vi "Field vs Slow IV v2.1.vi"() -> ()   [LabVIEW 2024]
uses:
  <vilib>/Utility/file.llb/Write Delimited Spreadsheet (DBL).vi
panel:
  in  "Tab Control 2":enum32{"cRIO", "Lockin", "Plot 2", "Plot 3"}(tab)
  out "I vs AI":cluster{"Y":dbl[], "Y":dbl[]}[](graph)
  out "Name 0":string="DC Voltage V"
  out "I vs R":cluster{"Y":dbl[], "Y":dbl[]}[](graph)
  out "Name 1":string="DC current uA"
  out "Name 2":string="dV V"
  out "Name 3":string="dI uA"
  in  "Tab Control":T1(tab)=enum."Data log and Status"
  in  "cRIO IP":string="//172.22.11.2"
  in  "Reading Average times":i32=100
  in  "Current Start uA":dbl=-1.5
  in  "Current Range uA":dbl=3.0
  in  "Current Step uA":dbl=0.005
  in  "Current output Scale factor":dbl=1.0
  in  "Ramp type":string(combo)="Range"
  in  "Ramp up first T":bool=TRUE
  in  "AO Channel":string(combo)="AO0"
  in  "Delay Time s":dbl=0.1 caption="Delay Time (s)"
  in  "Channel name 0":string(combo)="DC Voltage V"
  in  "Scale factor0":dbl=0.0001
  in  "Chan 1":bool=TRUE
  in  "Channel name 1":string(combo)="DC current uA"
  in  "Scale factor1":dbl=1.0
  in  "Chan 2":bool
  in  "Channel name 2":string(combo)="dV V"
  in  "Scale factor2":dbl=1.0
  in  "Chan 3":bool
  in  "Channel name 3":string(combo)="dI uA"
  in  "Scale factor3":dbl=1.0
  in  "Lockin Chan name 1":string(combo)="Voltage mV"
  in  "Lockin Chan name 2":string(combo)="Current mV"
  in  "Use Lockin":bool
  in  "Lockin 1":bool
  in  "Lockin 2":bool
  in  "Lockin address 1":string="GPIB0::8::INSTR"
  in  "Lockin address 2":string="GPIB0::9::INSTR"
  in  "Lockin Status":string
  in  "Contour plot folder":path=path "C:/Users/gyue/Desktop/20230814 Soorya devices"
  in  "Book name":string="book793"
  in  "Current VI path":path=path "C:/Users/gyue/Desktop/General-Measurement/cRIO related/Field vs Slow IV v2.1.vi"
  out "Current Field mT":dbl=8.0
  in  "stop":bool
  out "error out":errorcluster
  in  "Ramp up first T 2":bool=TRUE
  in  "Ramp type 2":string(combo)="Range"
  in  "Field Origin mT":dbl=-1.0 format="%#_13g"
  in  "Field step mT":dbl=0.1 format="%#_13g"
  in  "Field Radius mT":dbl=9.0 format="%#_13g"
  in  "Field Rate mT per sec":dbl=0.1 format="%#_13g"
  in  "Magnet Device Select":string(combo)="Elsa Magnet mT"
  # "Voltage x factor=uA"
  # "Voltage x factor=actual"
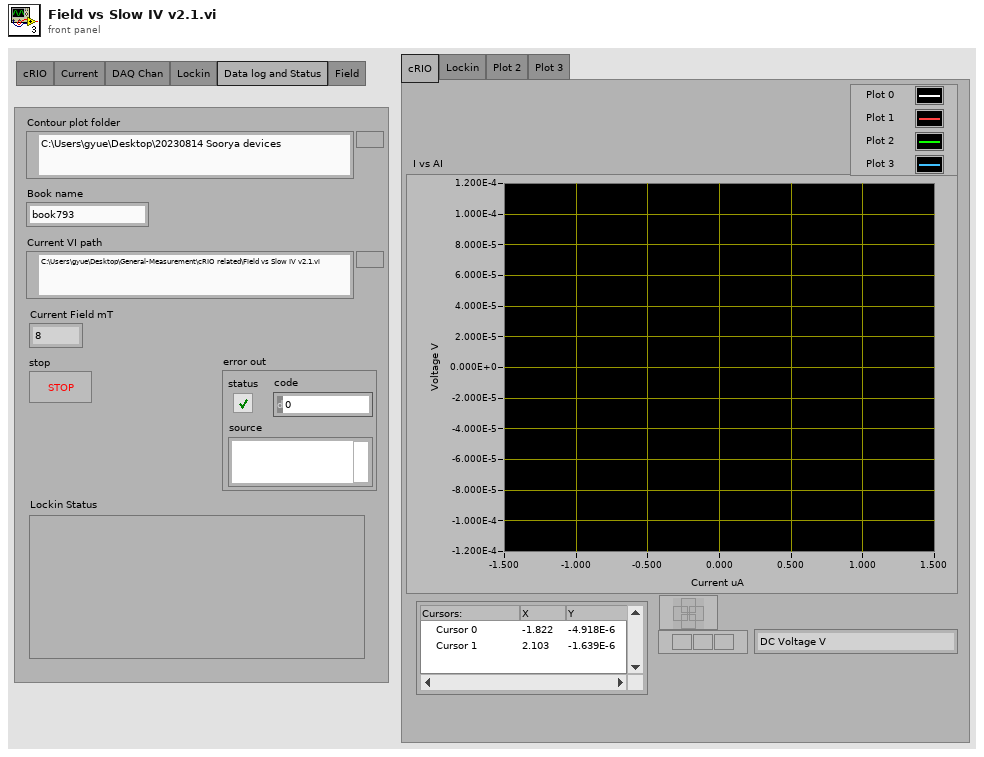
[diagram p1: front panel]
types:
  T1 = enum32{"cRIO", "Current", "DAQ Chan", "Lockin", "Data log and Status", "Field"}
  T2 = cluster{"AI0":dbl, "AI1":dbl, "AI2":dbl, "AI3":dbl}
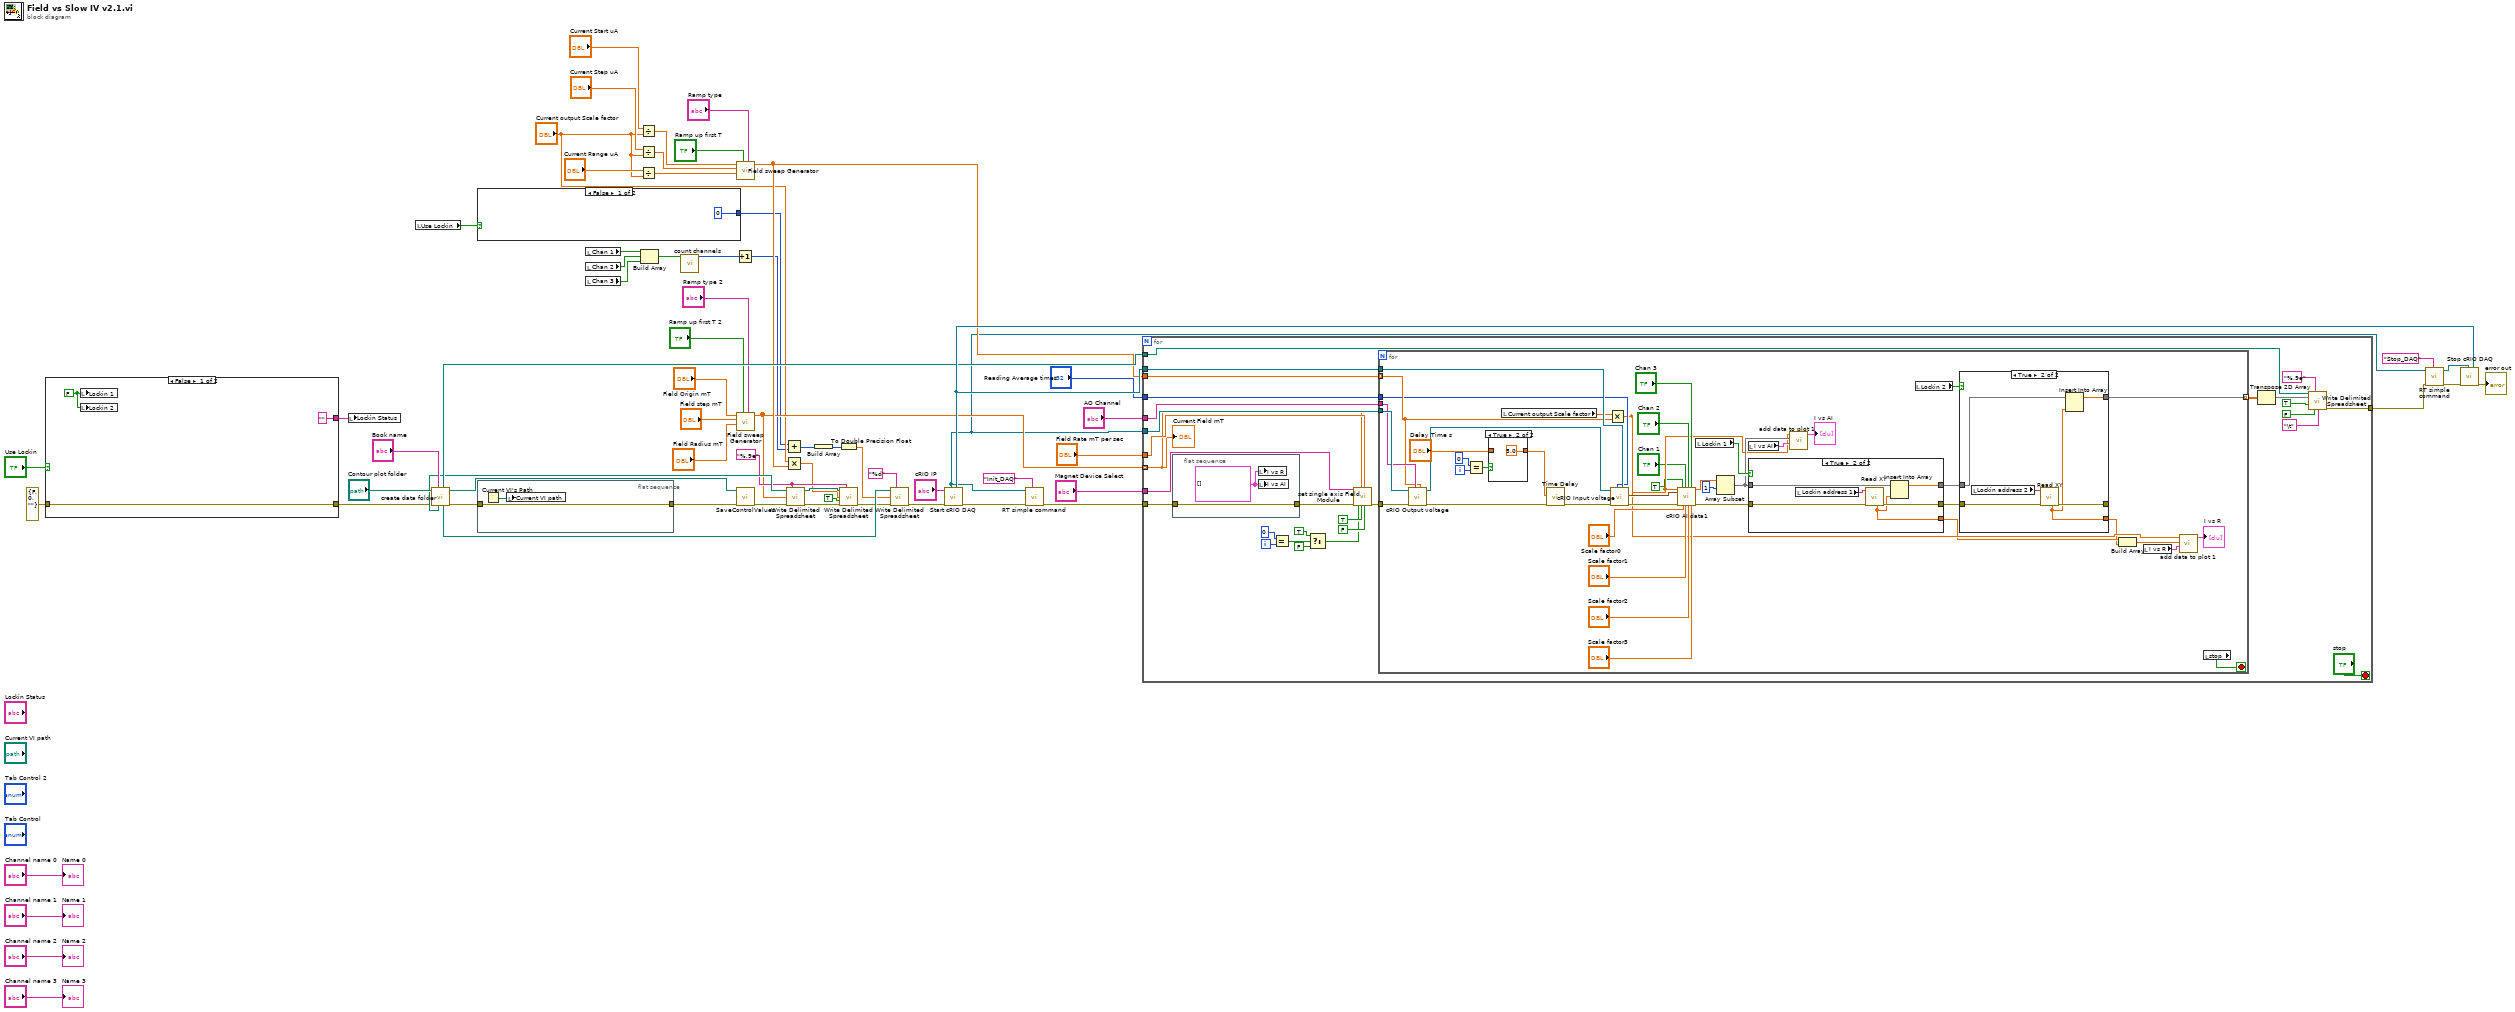
[diagram p0: block diagram]
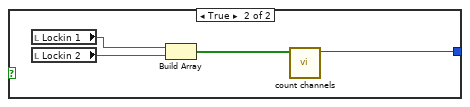
[diagram p2: hidden frame]
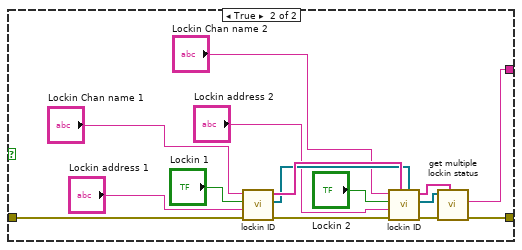
[diagram p3: hidden frame]
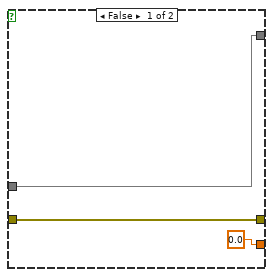
[diagram p4: hidden frame]
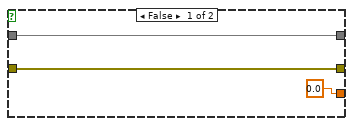
[diagram p5: hidden frame]
diagram:
  w38 = "%.9e" ("format (%.3f)")
  n1 = case shown="False" "Use Lockin" {
    tunnel: ["" ("Status output") w71] -> w15
    tunnel: [w70 w85] -> w14
    tunnel: errorcluster {"status"=FALSE, "code"=0, "source"=""} ("error in") -> [w70 w84]
    frame False {
      w68 = FALSE ("Lockin 1")
      n2 = local write "Lockin 1"(w68) -> ()
      n3 = local write "Lockin 2"(w68) -> ()
    }
    frame True {
      n4 = call "lockin ID.vi"("error in (no error)"=w84, "Lockin address"="Lockin address 1", "Lockin on"="Lockin 1", "Lockin Chan name"="Lockin Chan name 1") -> ("error out"=w83:errorcluster, "Addresses out"=w78:refnum<visa-resource-name>[], "names out"=w79:string[])  [unwired: 5 in]
      n5 = call "lockin ID.vi"("Addresses IN"=w78, "names in"=w79, "error in (no error)"=w83, "Lockin address"="Lockin address 2", "Lockin on"="Lockin 2", "Lockin Chan name"="Lockin Chan name 2") -> ("error out"=w72:errorcluster, "Addresses out"=w73:refnum<visa-resource-name>[], "names out"=w74:string[])  [unwired: 3 in]
      n6 = call "get multiple lockin status.vi"("Device channel names"=w74, "error in (no error)"=w72, "SRS830 addresses"=w73) -> ("error out"=w85:errorcluster, "Status output"=w71:string)  [unwired: 6 in, 1 out]
    }
  }
  n7 = local write "Lockin Status"(w15) -> ()
  n8 = local read "Use Lockin"() -> (w7:bool)
  n9 = call "create data folder.vi"("Book name"="Book name", "error in"=w14, "Contour plot folder"="Contour plot folder") -> ("error out"=w47:errorcluster, "xml path"=w49:path, "book par"=w32:path, "IV path"=w48:path, "Field path"=w45:path)  [unwired: 4 in]
  n10 = case shown="False" w7 {
    tunnel: [i16 0 ("x") w87] -> w6
    frame False {
    }
    frame True {
      n11 = local read "Lockin 1"() -> (w89:bool)
      n12 = local read "Lockin 2"() -> (w88:bool)
      n13 = Build Array(w89, w88) -> (w90:bool[])
      n14 = call "count channels.vi"("Array"=w90) -> ("Chan 3"=w87:i16)  [unwired: 10 in]
    }
  }
  n15 = flat-sequence {
    tunnel: w47 -> [w91]
    tunnel: [w91] -> w46
    frame #0 {
      n16 = Current VI's Path() -> (path=w92:path)
      n17 = local write "Current VI path"(w92) -> ()
    }
  }
  n18 = local read "Chan 1"() -> (w30:bool)
  n19 = local read "Chan 2"() -> (w29:bool)
  n20 = local read "Chan 3"() -> (w28:bool)
  n21 = Divide(x="Current Start uA", y="Current output Scale factor") -> (x/y=w61:dbl)
  n22 = Divide(x="Current Step uA", y="Current output Scale factor") -> (x/y=w60:dbl)
  n23 = Divide(x="Current Range uA", y="Current output Scale factor") -> (x/y=w59:dbl)
  n24 = Build Array(w30, w29, w28) -> (w27:bool[])
  n25 = call "count channels.vi"("Array"=w27) -> ("Chan 3"=w26:i16)  [unwired: 10 in]
  n26 = Increment(x=w26) -> (x+1=w9:i16)
  n27 = call "Field sweep Generator.vi"("Ramp type"="Ramp type", "Ramp up first T"="Ramp up first T", "Field Radius"=w59, "Field step"=w60, "Field Origin"=w61) -> ("output array"=w36:dbl[])  [unwired: 6 in]
  n28 = call "Field sweep Generator.vi"("Ramp type"="Ramp type 2", "Ramp up first T"="Ramp up first T 2", "Field Radius"="Field Radius mT", "Field step"="Field step mT", "Field Origin"="Field Origin mT") -> ("output array"=w22:dbl[])  [unwired: 6 in]
  n29 = call "SaveControlValues.vi"("XML File Path"=w49, "error in (no error)"=w46) -> ("error out"=w44:errorcluster)  [unwired: 8 in]
  n30 = Add(x=w6, y=w9) -> (x+y=w8:i16)
  n31 = Multiply(x="Current output Scale factor", y=w36) -> (x*y=w20:dbl[])
  n32 = call-poly <vilib>:"Write Delimited Spreadsheet.vi"("file path (dialog if empty)"=w45, "format (%.3f)"=w38, "1D data"=w22, "error in (no error)"=w44) -> ("new file path (Not A Path if cancelled)"=w37:path, "error out"=w34:errorcluster)  [unwired: 10 in]
  n33 = Build Array(w8) -> (w25:i16[])
  n34 = To Double Precision Float(number=w25) -> (double precision float=w24:dbl[])
  n35 = call-poly <vilib>:"Write Delimited Spreadsheet.vi"("file path (dialog if empty)"=w37, "format (%.3f)"=w38, "1D data"=w20, "append to file? (new file:F)"=TRUE, "error in (no error)"=w34) -> ("error out"=w31:errorcluster)  [unwired: 9 in, 1 out]
  n36 = call-poly <vilib>:"Write Delimited Spreadsheet.vi"("file path (dialog if empty)"=w32, "format (%.3f)"="%d", "1D data"=w24, "error in (no error)"=w31) -> ("error out"=w23:errorcluster)  [unwired: 10 in, 1 out]
  n37 = call "Start cRIO DAQ.vi"("error in (no error)"=w23, "cRIO IP"="cRIO IP") -> ("error out"=w11:errorcluster, "DAQ_AI_Reader endpoint"=w57:refnum<k21>, "DAQ_CMD_Writer endpoint"=w4:refnum<k21>)  [unwired: 7 in]
  n38 = call "RT simple command.vi"("Command"="Init_DAQ", "error in (no error)"=w11, "DAQ_CMD_Writer endpoint"=w4) -> ("error out"=w10:errorcluster)  [unwired: 7 in, 1 out]
  n39 = for {
    tunnel: "AO Channel" -> [w120]
    tunnel: w36 -> [w119]
    tunnel: w4 -> [w118]
    tunnel: w57 -> [w117]
    tunnel: "Reading Average times" -> [w116]
    tunnel: w48 -> [w111]
    tunnel: w22 -> [w113] mode=indexing
    tunnel: w10 -> [w94]
    tunnel: [w106] -> w3
    tunnel: "Field Rate mT per sec" -> [w114]
    tunnel: "Magnet Device Select" -> [w96]
    i -> [w102]
    stop <- "stop" stop-if-true
    n40 = flat-sequence {
      tunnel: w94 -> [w122]
      tunnel: [w122] -> w93
      frame #0 {
        w121 = cluster{dbl[], dbl[]}[] []
        n41 = local write "I vs R"(w121) -> ()
        n42 = local write "I vs AI"(w121) -> ()
      }
    }
    n43 = Equal?(x=0, y=w102) -> (x = y?=w100:bool)
    n44 = Select(t=TRUE ("Init"), s=w100, f=FALSE) -> (s? t:f=w97:bool)
    n45 = call "set single axis Field Module.vi"("Field Device Select"=w96, "error in (no error)"=w93, "Init"=w97, "Field Target mT or dBm"=w113, "Exec"=TRUE, "Field Rate mT per sec"=w114, "final"=FALSE) -> ("error out"=w112:errorcluster)  [unwired: 12 in]
    n46 = for {
      tunnel: w112 -> [w165]
      tunnel: w118 -> [w164]
      tunnel: w120 -> [w163]
      tunnel: w119 -> [w157] mode=indexing
      tunnel: w117 -> [w161]
      tunnel: w116 -> [w156]
      tunnel: [w131] -> w105 mode=indexing
      i -> [w153]
      stop <- w149 stop-if-true
      n47 = call "cRIO Output voltage.vi"("Voltage"=w157, "AO Channel"=w163, "error in (no error)"=w165, "DAQ_CMD_Writer endpoint"=w164) -> ("error out"=w160:errorcluster, "DAQ_CMD_Writer endpoint out"=w162:refnum<k21>)  [unwired: 6 in]
      n48 = Equal?(x=0, y=w153) -> (x = y?=w152:bool)
      n49 = case shown="True" w152 {
        tunnel: "Delay Time s" -> [w184 _]
        tunnel: [w184 5.0 ("Delay Time s")] -> w150
        frame False {
        }
        frame True {
        }
      }
      n50 = local read "Current output Scale factor"() -> (w158:dbl)
      n51 = call "Time Delay"("error in (no error)"=w160, "Delay Time (s)"=w150) -> ("error out"=w159:errorcluster)  [unwired: 9 in]
      n52 = Multiply(x=w158, y=w157) -> (x*y=w129:dbl)
      n53 = call "cRIO Input voltage.vi"("DAQ_AI_Reader endpoint"=w161, "Average"=w156, "error in (no error)"=w159, "DAQ_CMD_Writer endpoint"=w162) -> ("error out"=w148:errorcluster, "output cluster"=w141:T2)  [unwired: 5 in, 1 out]
      n54 = call "cRIO AI data1.vi"("I"=w129, "Input cluster"=w141, "error in (no error)"=w148, "Chan 0"=TRUE, "Scale factor0"="Scale factor0", "Chan 1"="Chan 1", "Scale factor1"="Scale factor1", "Chan 2"="Chan 2", "Scale factor2"="Scale factor2", "Chan 3"="Chan 3", "Scale factor3"="Scale factor3") -> ("Output data"=w139:dbl[], "error out"=w135:errorcluster)  [unwired: 7 in]
      n55 = local read "Lockin 1"() -> (w137:bool)
      n56 = Array Subset(array=w139, index=1) -> (w136:dbl[])  [unwired: 1 in]
      n57 = local read "I vs AI"() -> (w140:cluster{"Y":dbl[], "Y":dbl[]}[])
      n58 = case shown="True" w137 {
        tunnel: w135 -> [w176 w182]
        tunnel: [w176 w179] -> w134
        tunnel: w136 -> [w177 w181]
        tunnel: [w177 w180] -> w132
        tunnel: [0.0 ("R") w178] -> w128
        frame False {
        }
        frame True {
          n59 = local read "Lockin address 1"() -> (w183:string)
          n60 = call "Read XY.vi"("error in (no error)"=w182, "VISA resource name"=w183) -> ("error out"=w179:errorcluster, "R"=w178:dbl)  [unwired: 5 in, 3 out]
          n61 = Insert Into Array(array=w181, new element=w178) -> (w180:dbl[])  [unwired: 1 in]
        }
      }
      n62 = call "add data to plot 1.vi"("Input graph"=w140, "Input Y array"=w136, "x"=w129) -> ("Output graph"=→"I vs AI":cluster{dbl[], dbl[]}[])  [unwired: 7 in, 1 out]
      n63 = local read "Lockin 2"() -> (w133:bool)
      n64 = case shown="True" w133 {
        tunnel: w134 -> [w167 w173]
        tunnel: [w167 w170] -> _
        tunnel: w132 -> [w168 w172]
        tunnel: [w168 w171] -> w131
        tunnel: [0.0 ("R") w169] -> w127
        frame False {
        }
        frame True {
          n65 = local read "Lockin address 2"() -> (w174:string)
          n66 = call "Read XY.vi"("error in (no error)"=w173, "VISA resource name"=w174) -> ("error out"=w170:errorcluster, "R"=w169:dbl)  [unwired: 5 in, 3 out]
          n67 = Insert Into Array(array=w172, new element=w169) -> (w171:dbl[])  [unwired: 1 in]
        }
      }
      n68 = Build Array(w128, w127) -> (w126:dbl[])
      n69 = local read "I vs R"() -> (w130:cluster{"Y":dbl[], "Y":dbl[]}[])
      n70 = call "add data to plot 1.vi"("Input graph"=w130, "Input Y array"=w126, "x"=w129) -> ("Output graph"=→"I vs R":cluster{dbl[], dbl[]}[])  [unwired: 7 in, 1 out]
      n71 = local read "stop"() -> (w149:bool)
    }
    n72 = Transpose 2D Array(2D array=w105) -> (transposed array=w95:dbl[][])
    n73 = call-poly <vilib>:"Write Delimited Spreadsheet.vi"("file path (dialog if empty)"=w111, "format (%.3f)"="%.9e", "2D data"=w95, "append to file? (new file:F)"=TRUE, "transpose? (no:F)"=FALSE, "delimiter (\\t)"="\t" ("delimiter (\\t)")) -> ("error out"=w106:errorcluster)  [unwired: 8 in, 1 out]
    "Current Field mT" <- w113
  }
  n74 = call "RT simple command.vi"("Command"="Stop_DAQ", "error in (no error)"=w3, "DAQ_CMD_Writer endpoint"=w4) -> ("error out"=w2:errorcluster, "DAQ_CMD_Writer endpoint out"=w1:refnum<k21>)  [unwired: 7 in]
  n75 = call "Stop cRIO DAQ.vi"("DAQ_AI_Reader endpoint"=w57, "DAQ_CMD_Writer endpoint"=w1, "error in (no error)"=w2) -> ("error out"=→"error out":errorcluster)  [unwired: 8 in]
  "Name 0" <- "Channel name 0"
  "Name 1" <- "Channel name 1"
  "Name 2" <- "Channel name 2"
  "Name 3" <- "Channel name 3"
